vi "Send Batch Messages To Specific Target.vi"(8 "error in (no error)":errorcluster, 9 "Mail Strategy In":refnum<class "Mail Strategy.lvclass">, 10 "Messages In":refnum<class "Message.lvclass">[](array[class]), 11 "Messenger in":refnum<class "Tree-ArrayLocation Queue Messenger.lvclass">) -> (0 "error out":errorcluster, 3 "Messenger out":refnum<class "Tree-ArrayLocation Queue Messenger.lvclass">)   [LabVIEW 2019, in "Tree-ArrayLocation Queue Messenger.lvclass"]
uses:
  Tree-ArrayLocation Queue Messenger.lvclass
  C:/Users/iio/Desktop/NTHU Brain Center/General Purpose/Classes/Ancestor/Messenger/Messenger Composite/Messenger Composite.lvclass
  Ancestor Class/Message/Message.lvclass
  Ancestor Class/Messenger/Mail Strategy/Mail Strategy.lvclass
  Array Location Mailman/Array Location Mailman.lvclass
  C:/Users/iio/Desktop/NTHU Brain Center/General Purpose/Classes/Ancestor/Messenger/Mail Strategy/Mail Strategy.lvclass
  Array Location Mailman/Array Location Mailman.lvclass/Array Location Mailman.ctl
  Ancestor Class/Messenger/Messenger Composite/Messenger Composite.lvclass/Messenger Composite.ctl
  Tree-ArrayLocation Queue Messenger.lvclass/Tree-ArrayLocation Queue Messenger.ctl
  Array Location Mailman/Public Data/Write Location.vi
  Ancestor Class/Messenger/Messenger Composite/Public Data/Read Nodes.vi
  Array Location Mailman/Public Data/Read Location.vi
  Ancestor Class/Messenger/Messenger/Messenger.lvclass
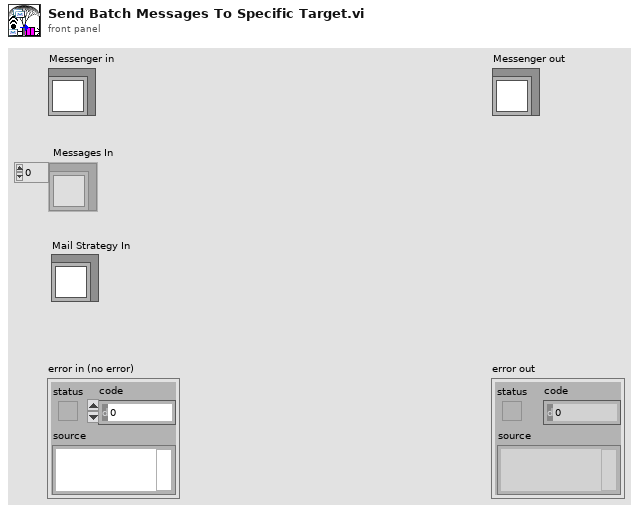
[diagram p1: front panel]
types:
  T1 = typedef "Message Queue.ctl" = refnum<queue>
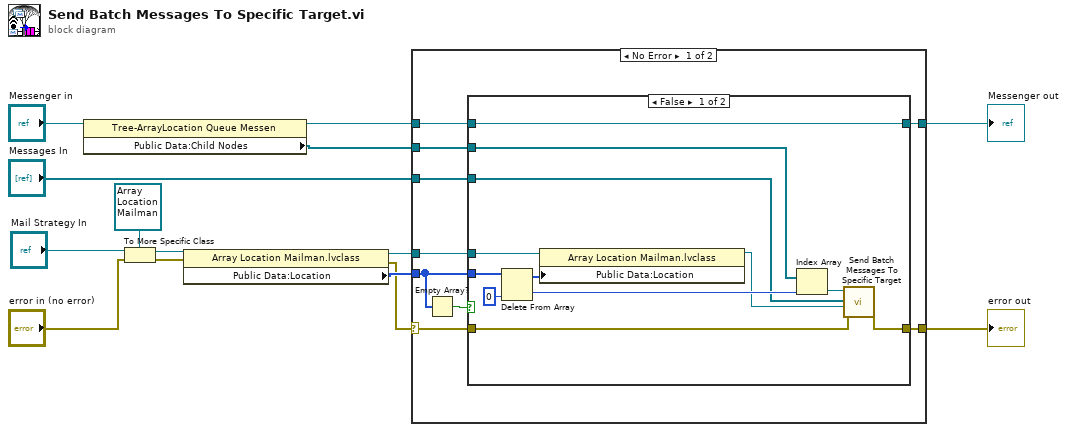
[diagram p0: block diagram]
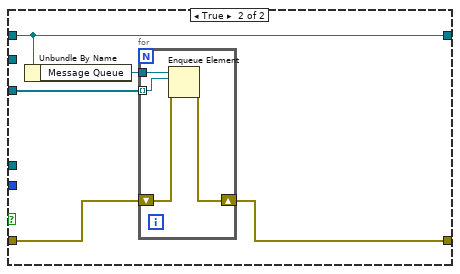
[diagram p2: hidden frame]
diagram:
  n1 = property class="Tree-ArrayLocation Queue Messen"(reference="Messenger in") -> (reference out=w3:refnum<class "Tree-ArrayLocation Queue Messenger.lvclass">, "Public Data:Child Nodes"=w2:refnum<class "Messenger.lvclass">[])  [unwired: 1 in, 1 out]
  n2 = To More Specific Class(target class=refnum<class "Array Location Mailman.lvclass"> refnum ("Array Location Mailman.lvclass"), reference="Mail Strategy In", error in="error in (no error)") -> (specific class reference=w8:refnum<class "Array Location Mailman.lvclass">, error out=w9:errorcluster)
  n3 = property class="Array Location Mailman.lvclass"(reference=w8, error in=w9) -> (reference out=w1:refnum<class "Array Location Mailman.lvclass">, error out=w6:errorcluster, "Public Data:Location"=w7:i32[])
  n4 = case shown="No Error" w6 {
    selector: w6 -> [w18 w45]
    tunnel: w3 -> [w22 w46]
    tunnel: [w20 w46] -> w14
    tunnel: [w17 w45] -> w13
    tunnel: w7 -> [w19 _]
    tunnel: "Messages In" -> [w21 _]
    tunnel: w2 -> [w16 _]
    tunnel: w1 -> [w15 _]
    frame No Error {
      n5 = Empty Array?(array=w19) -> (empty?=w23:bool)
      n6 = case shown="False" w23 {
        tunnel: w22 -> [w35 w40]
        tunnel: w21 -> [w28 w38]
        tunnel: [w35 w40] -> w20
        tunnel: w19 -> [w34 _]
        tunnel: w18 -> [w30 w37]
        tunnel: [w29 w36] -> w17
        tunnel: w16 -> [w27 _]
        tunnel: w15 -> [w26 _]
        frame False {
          n7 = Delete From Array(array=w34, index=0) -> (deleted portion=w32:i32, array with subset deleted=w25:i32[])  [unwired: 1 in]
          n8 = property class="Array Location Mailman.lvclass"(reference=w26, "Public Data:Location"=w25) -> (reference out=w24:refnum<class "Array Location Mailman.lvclass">)  [unwired: 1 in, 1 out]
          n9 = Index Array(array=w27, index=w32) -> (element=w31:refnum<class "Messenger.lvclass">)
          n10 = call-dynamic "Send Batch Messages To Specific Target.vi"("error in (no error)"=w30, "Mail Strategy In"=w24, "Messages In"=w28, "Messenger in"=w31) -> ("error out"=w29:errorcluster)  [unwired: 6 in, 1 out]
        }
        frame True {
          n11 = Unbundle By Name(w40) -> ("Message Queue"=w39:T1)
          n12 = for {
            tunnel: w39 -> [w44]
            tunnel: w38 -> [w43] mode=indexing
            shift-right: [w41] -> w36
            shift-left: w37 -> [w42]
            n13 = Enqueue Element(queue=w44, element=w43, error in (no error)=w42) -> (error out=w41:errorcluster)  [unwired: 1 in, 2 out]
          }
        }
      }
    }
    frame Error {
    }
  }
  "error out" <- w13
  "Messenger out" <- w14
